vi "Button logic.vi"(11 "Secondary":T1) -> (3 "RPM Set":dbl)   [LabVIEW 2012]
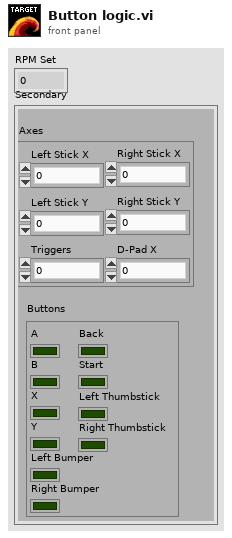
[diagram p1: front panel]
types:
  T1 = cluster{"Buttons":cluster{"A":bool, "B":bool, "X":bool, "Y":bool, "Left Bumper":bool, "Right Bumper":bool, "Back":bool, "Start":bool, "Left Thumbstick":bool, "Right Thumbstick":bool}, "Axes":cluster{"Left Stick X ":dbl, "Left Stick Y":dbl, "Triggers":dbl, "Right Stick X":dbl, "Right Stick Y":dbl, "D-Pad X":dbl}}
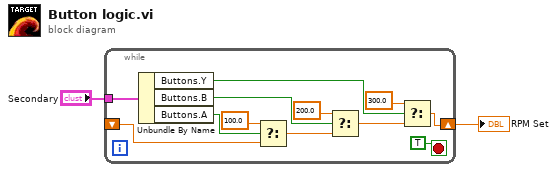
[diagram p0: block diagram]
diagram:
  n1 = while {
    shift-right: [w8] -> w1
    shift-left: _ -> [w9]
    tunnel: "Secondary" -> [w6]
    stop <- TRUE stop-if-true
    n2 = Unbundle By Name(w6) -> ("Buttons.Y"=w5:bool, "Buttons.B"=w4:bool, "Buttons.A"=w3:bool)
    n3 = Select(t=100.0, s=w3, f=w9) -> (s? t:f=w13:dbl)
    n4 = Select(t=200.0, s=w4, f=w13) -> (s? t:f=w11:dbl)
    n5 = Select(t=300.0, s=w5, f=w11) -> (s? t:f=w8:dbl)
  }
  "RPM Set" <- w1
